vi "bulk Write Tx Only.vi"(8 "error in (no error)":errorcluster, 9 "param_length":u16, 10 "protocol_version":i32, 11 "port_num":i32) -> (0 "error out":errorcluster)   [LabVIEW 2018, in "labview.lvlib"]
doc: "WINDECLSPEC void bulkWriteTxOnly (int port_num, int protocol_version, uint16_t param_length);"
uses:
  labview.lvlib
  dxl_x86_c.dll
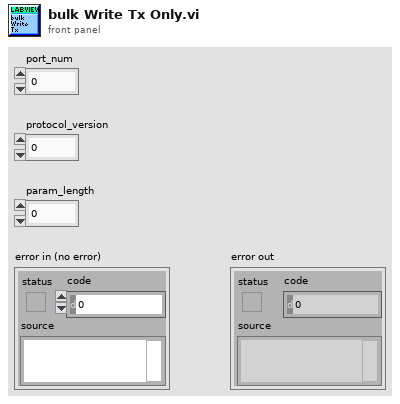
[diagram p1: front panel]
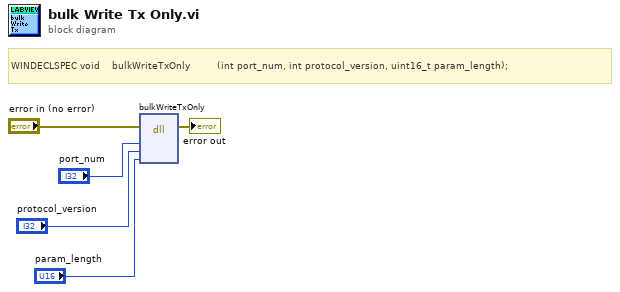
[diagram p0: block diagram]
diagram:
  # "WINDECLSPEC void    bulkWriteTxOnly         (int port_num, int protocol_version, uint16_t param_length);"
  n1 = dll-call lib="C:/Users/joaos/OneDrive/Documents/[PhD]/Project Omnidirectional Vehicle/Vanes/LabView_code/joaoandthethreestands/DynamixelSDK-3.7.31/labview/new_compilation/dxl_x86_c.*" fn="bulkWriteTxOnly"(error in="error in (no error)", "port_num"="port_num", "protocol_version"="protocol_version", "param_length"="param_length") -> (error out=→"error out":errorcluster)  [unwired: 6 in, 1 out]
